vi "获取数据.vi"(11 "table":string) -> (3 "输出簇":T1)   [LabVIEW 2016, in "DGUS.lvlib"]
uses:
  DGUS.lvlib
  PLC/PLC.lvlib
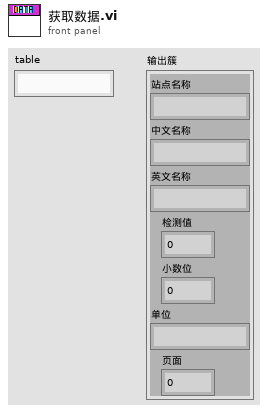
[diagram p1: front panel]
types:
  T1 = cluster{"站点名称":string, "中文名称":string, "英文名称":string, "检测值":sgl, "小数位":u8, "单位":string, "页面":u16}
  T2 = cluster{"AD0":sgl, "AD1":sgl, "AD2":sgl, "AD3":sgl, "AD4":sgl, "AD5":sgl}
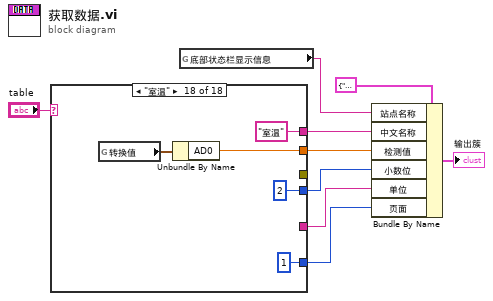
[diagram p0: block diagram]
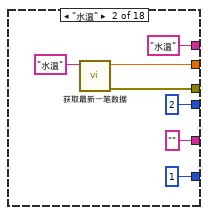
[diagram p3: hidden frame]
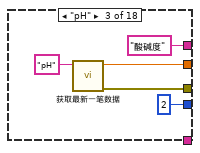
[diagram p4: hidden frame]
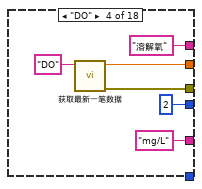
[diagram p5: hidden frame]
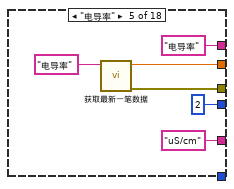
[diagram p6: hidden frame]
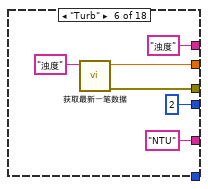
[diagram p7: hidden frame]
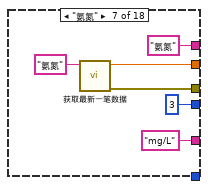
[diagram p8: hidden frame]
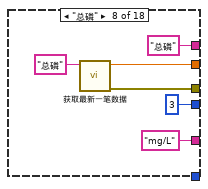
[diagram p9: hidden frame]
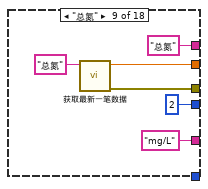
[diagram p10: hidden frame]
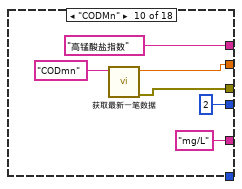
[diagram p11: hidden frame]
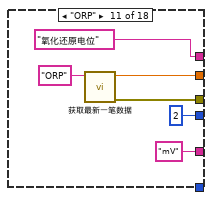
[diagram p12: hidden frame]
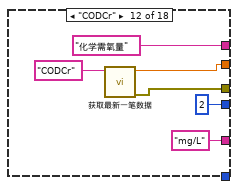
[diagram p13: hidden frame]
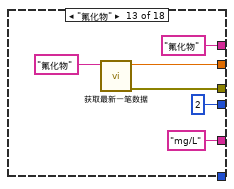
[diagram p14: hidden frame]
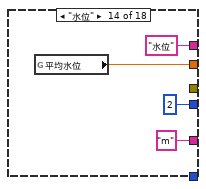
[diagram p15: hidden frame]
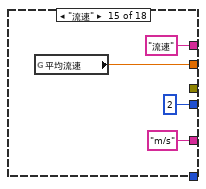
[diagram p16: hidden frame]
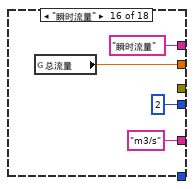
[diagram p17: hidden frame]
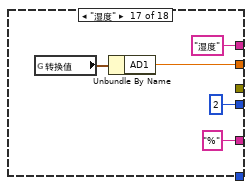
[diagram p18: hidden frame]
diagram:
  n1 = case shown="\"室温\"" "table" {
    tunnel: [_ w16 w21 w27 w33 w39 w45 w51 w57 w63 w69 w75 w81 _ _ _ _ _] -> _
    tunnel: [_ "水温" ("显示参数中文名") "酸碱度" ("显示参数中文名") "溶解氧" ("显示参数中文名") "电导率" ("显示参数中文名") "浊度" ("显示参数中文名") "氨氮" ("显示参数中文名") "总磷" ("显示参数中文名") "总氮" ("显示参数中文名") "高锰酸盐指数" ("显示参数中文名") "氧化还原电位" ("显示参数中文名") "化学需氧量" ("显示参数中文名") "氟化物" ("显示参数中文名") "水位" ("显示参数中文名") "流速" ("显示参数中文名") "瞬时流量" ("显示参数中文名") "湿度" ("显示参数中文名") "室温" ("显示参数中文名")] -> w6
    tunnel: [_ "" ("显示单位") _ "mg/L" ("显示单位") "uS/cm" ("显示单位") "NTU" ("显示单位") "mg/L" ("显示单位") "mg/L" ("显示单位") "mg/L" ("显示单位") "mg/L" ("显示单位") "mV" ("显示单位") "mg/L" ("显示单位") "mg/L" ("显示单位") "m" ("显示单位") "m/s" ("显示单位") "m3/s" ("显示单位") "%" ("显示单位") _] -> w5
    tunnel: [_ u8 2 ("小数位") u8 2 ("小数位") u8 2 ("小数位") u8 2 ("小数位") u8 2 ("小数位") u8 3 ("小数位") u8 3 ("小数位") u8 2 ("小数位") u8 2 ("小数位") u8 2 ("小数位") u8 2 ("小数位") u8 2 ("小数位") u8 2 ("小数位") u8 2 ("小数位") u8 2 ("小数位") u8 2 ("小数位") u8 2 ("小数位")] -> w4
    tunnel: [_ u16 1 ("页面") _ _ _ _ _ _ _ _ _ _ _ _ _ _ _ u16 1 ("页面")] -> w3
    tunnel: [_ w10 w18 w22 w30 w36 w40 w48 w52 w60 w64 w72 w77 w83 w88 w92 w96 w101] -> w2
    frame Default {
    }
    frame "水温" {
      n2 = call "获取最新一笔数据.vi"("table"="水温") -> ("错误输出"=w16:errorcluster, "data"=w10:dbl)  [unwired: 8 in, 1 out]
    }
    frame "pH" {
      n3 = call "获取最新一笔数据.vi"("table"="pH") -> ("错误输出"=w21:errorcluster, "data"=w18:dbl)  [unwired: 8 in, 1 out]
    }
    frame "DO" {
      n4 = call "获取最新一笔数据.vi"("table"="DO") -> ("错误输出"=w27:errorcluster, "data"=w22:dbl)  [unwired: 8 in, 1 out]
    }
    frame "电导率" {
      n5 = call "获取最新一笔数据.vi"("table"="电导率") -> ("错误输出"=w33:errorcluster, "data"=w30:dbl)  [unwired: 8 in, 1 out]
    }
    frame "Turb" {
      n6 = call "获取最新一笔数据.vi"("table"="浊度") -> ("错误输出"=w39:errorcluster, "data"=w36:dbl)  [unwired: 8 in, 1 out]
    }
    frame "氨氮" {
      n7 = call "获取最新一笔数据.vi"("table"="氨氮") -> ("错误输出"=w45:errorcluster, "data"=w40:dbl)  [unwired: 8 in, 1 out]
    }
    frame "总磷" {
      n8 = call "获取最新一笔数据.vi"("table"="总磷") -> ("错误输出"=w51:errorcluster, "data"=w48:dbl)  [unwired: 8 in, 1 out]
    }
    frame "总氮" {
      n9 = call "获取最新一笔数据.vi"("table"="总氮") -> ("错误输出"=w57:errorcluster, "data"=w52:dbl)  [unwired: 8 in, 1 out]
    }
    frame "CODMn" {
      n10 = call "获取最新一笔数据.vi"("table"="CODmn") -> ("错误输出"=w63:errorcluster, "data"=w60:dbl)  [unwired: 8 in, 1 out]
    }
    frame "ORP" {
      n11 = call "获取最新一笔数据.vi"("table"="ORP") -> ("错误输出"=w69:errorcluster, "data"=w64:dbl)  [unwired: 8 in, 1 out]
    }
    frame "CODCr" {
      n12 = call "获取最新一笔数据.vi"("table"="CODCr") -> ("错误输出"=w75:errorcluster, "data"=w72:dbl)  [unwired: 8 in, 1 out]
    }
    frame "氟化物" {
      n13 = call "获取最新一笔数据.vi"("table"="氟化物") -> ("错误输出"=w81:errorcluster, "data"=w77:dbl)  [unwired: 8 in, 1 out]
    }
    frame "水位" {
      n14 = global read "流量计全局变量.vi" "平均水位"() -> (w83:dbl)
    }
    frame "流速" {
      n15 = global read "流量计全局变量.vi" "平均流速"() -> (w88:dbl)
    }
    frame "瞬时流量" {
      n16 = global read "流量计全局变量.vi" "总流量"() -> (w92:dbl)
    }
    frame "湿度" {
      n17 = global read "采配水全局变量.vi" "转换值"() -> (w98:T2)
      n18 = Unbundle By Name(w98) -> ("AD1"=w96:sgl)
    }
    frame "室温" {
      n19 = global read "采配水全局变量.vi" "转换值"() -> (w103:T2)
      n20 = Unbundle By Name(w103) -> ("AD0"=w101:sgl)
    }
  }
  n21 = global read "副屏设置全局变量.vi" "底部状态栏显示信息"() -> (w8:string)
  n22 = Bundle By Name(cluster=T1 {"站点名称"="", "中文名称"="", "英文名称"="", "检测值"=0.0, "小数位"=0, "单位"="", "页面"=0} ("data"), "站点名称"=w8, "中文名称"=w6, "检测值"=w2, "小数位"=w4, "单位"=w5, "页面"=w3) -> (→"输出簇":T1)
